vi "fpga_project_stable.vi"() -> ()   [LabVIEW 2019]
uses:
  <vilib>/Platform/TimedLoop/XDataNode/timing_clust.ctl
  <vilib>/Platform/TimedLoop/XDataNode/nitl_modes.ctl
  <vilib>/Platform/TimedLoop/XDataNode/wakeup.ctl
  <vilib>/rvi/eio/common/nirviEmuTemplateMethod_errors.vi
  <vilib>/rvi/Emulation/niFpgaSctlEmulationGetInTimedLoop.vi
  <vilib>/rvi/Emulation/niFpgaEmulationReportErrorSimple.vi
  <vilib>/rvi/Emulation/niFpgaGetClockAttributes.vi
  <vilib>/rvi/Emulation/niFpgaCriticalErrorInLSC.vi
  <vilib>/eio/EIONode/EIONode.xnode
  <vilib>/eio/EIOMethodNode/EIOMethodNode.xnode
  <vilib>/platform/TimedLoop/XDataNode/XDataNode.xnode
  <vilib>/Platform/TimedLoop/XDataNode/XDNodeRunTimeDep.lvlib
panel:
  out "SDA":bool
  out "ACK":bool
  in  "add + read bite":u8 format="%x"
  in  "register":u8 format="%x"
  in  "adresse + Write":u8 format="%x"
  out "adress + READ":bool[](array[boolean])
  out "DATA":u8 format="%b"
  out "DATA":bool[](array[boolean])
  out "register adress":bool[](array[boolean])
  out "Adresse + command byte":bool[](array[boolean])
  # "51"
  # "50"
  # "expected data :"
  # "00110011"
  # "15"
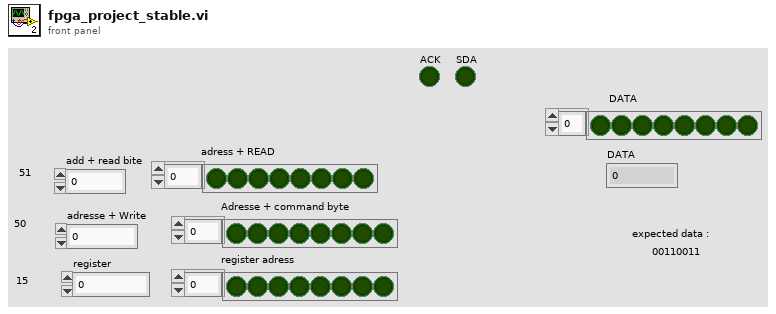
[diagram p1: front panel]
types:
  T1 = typedef "XDNodeRunTimeDep.lvlib/timing_clust.ctl" = cluster{"Expected End [f-1]":u64, "Actual End [f-1]":u64, "Finished Late? [f-1]":bool, "Expected End [i-1]":u64, "Actual End [i-1]":u64, "Finished Late? [i-1]":bool, "Expected Start [i]":u64, "Actual Start [i]":u64, "Expected Start [f]":u64, "Actual Start [f]":u64, "Source Name":string, "Structure Name":string, "Period":i64, "Deadline":i64, "Offset":i64, "Start":i64, "Priority":i32, "Timeout":i32, "Mode":T2, "Wakeup Reason":T3, "Error":errorcluster, "Source Type":string, "Secondary Source Type":string, "Global End Time":u64, "Global Start Time":u64, "Frame Duration":u64, "Iteration Duration":u64, "Assigned CPU":i32, "I/O Scan Engine Mode":u32}
  T2 = typedef "XDNodeRunTimeDep.lvlib/nitl_modes.ctl" = enum32{"No Change", "Process missed periods, maintain original phase", "Discard missed periods, maintain original phase", "Process missed periods, ignore original phase", "Discard missed periods, ignore original phase"}
  T3 = typedef "XDNodeRunTimeDep.lvlib/wakeup.ctl" = enum32{"Normal", "Aborted", "Asynchronous wakeup", "Timing source error", "Timed loop error", "Timeout"}
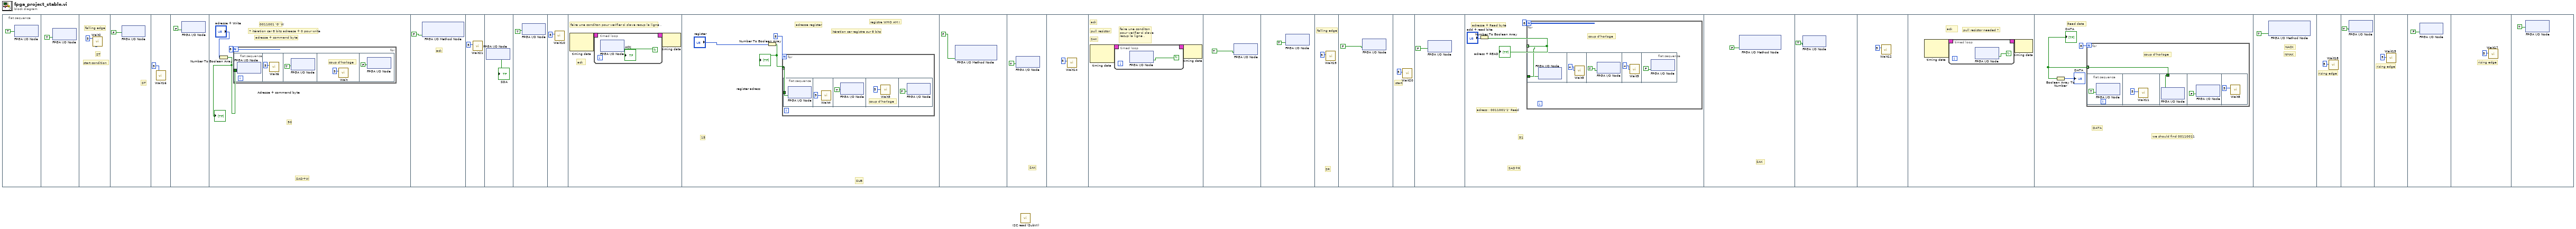
[diagram p0: block diagram]
diagram:
  n1 = flat-sequence {
    frame #0 {
      n2 = xnode "FPGA I/O Node"("SDA"=TRUE) -> ()  [unwired: 1 in, 1 out]
    }
    frame #1 {
      n3 = xnode "FPGA I/O Node"("SCL"=TRUE) -> ()  [unwired: 1 in, 1 out]
    }
    frame #2 {
      # "ST"
      # "start condition"
      # "falling edge"
      n4 = call "Wait2"("Count(Ticks)"=u32 5) -> ()  [unwired: 1 out]
    }
    frame #3 {
      # "ST"
      n5 = xnode "FPGA I/O Node"("SDA"=FALSE) -> ()  [unwired: 1 in, 1 out]
    }
    frame #4 {
      n6 = call "Wait16"("Count(Ticks)"=u32 5) -> ()  [unwired: 1 out]
    }
    frame #5 {
      n7 = xnode "FPGA I/O Node"("SCL"=FALSE) -> ()  [unwired: 1 in, 1 out]
    }
    frame #6 {
      # "50"
      # "SAD+W"
      # "7 itération car 8 bits adreese + 0 pour write"
      # "0011001 '0' W"
      # "adresse + command byte"
      n8 = Number To Boolean Array(number="adresse + Write") -> (Boolean array=w8:bool[])
      "Adresse + command byte" <- w8
      n9 = for {
        N: 8 -> [_]
        tunnel: w8 -> [w10] mode=indexing
        n10 = flat-sequence {
          tunnel: w10 -> [w11]
          frame #0 {
            n11 = xnode "FPGA I/O Node"("SDA"=w11) -> ()  [unwired: 1 in, 1 out]
          }
          frame #1 {
            n12 = call "Wait6"("Count(Ticks)"=u32 5) -> ()  [unwired: 1 out]
          }
          frame #2 {
            n13 = xnode "FPGA I/O Node"("SCL"=TRUE) -> ()  [unwired: 1 in, 1 out]
          }
          frame #3 {
            # "coup d'horloge"
            n14 = call "Wait"("Count(Ticks)"=u32 5) -> ()  [unwired: 1 out]
          }
          frame #4 {
            n15 = xnode "FPGA I/O Node"("SCL"=FALSE) -> ()  [unwired: 1 in, 1 out]
          }
        }
      }
    }
    frame #7 {
      # "ack"
      n16 = xnode "FPGA I/O Method Node"("Enable"=FALSE) -> ()  [unwired: 1 in, 1 out]
    }
    frame #8 {
      n17 = call "Wait21"("Count(Ticks)"=u32 5) -> ()  [unwired: 1 out]
    }
    frame #9 {
      n18 = xnode "FPGA I/O Node"() -> ("SDA"=→"SDA":bool)  [unwired: 1 in, 1 out]
    }
    frame #10 {
      n19 = xnode "FPGA I/O Node"("SCL"=TRUE) -> ()  [unwired: 1 in, 1 out]
    }
    frame #11 {
      n20 = call "Wait10"("Count(Ticks)"=u32 5) -> ()  [unwired: 1 out]
    }
    frame #12 {
      # "ack"
      # "faire une conditon pour verifier si slave recup la ligne ."
      n21 = node-c288() -> (w22:T1)  [unwired: 2 in]
      n22 = timed-loop {
        timing: w22 -> [_]
        timing-out: [_] -> w21
        stop <- w23 continue-if-true
        n23 = xnode "FPGA I/O Node"() -> ("SDA"=w23:bool)  [unwired: 1 in, 1 out]
        "ACK" <- w23
      }
      n24 = node-c288(w21) -> ()  [unwired: 1 out]
    }
    frame #13 {
      # "15"
      # "registre WHO AM I"
      # "itération car registre sur 8 bits"
      # "SUB"
      # "adresse register"
      n25 = Number To Boolean Array(number="register") -> (Boolean array=w30:bool[])
      "register adress" <- w30
      n26 = for {
        N: 8 -> [_]
        tunnel: w30 -> [w31] mode=indexing
        n27 = flat-sequence {
          tunnel: w31 -> [w32]
          frame #0 {
            n28 = xnode "FPGA I/O Node"("SDA"=w32) -> ()  [unwired: 1 in, 1 out]
          }
          frame #1 {
            n29 = call "Wait4"("Count(Ticks)"=u32 5) -> ()  [unwired: 1 out]
          }
          frame #2 {
            n30 = xnode "FPGA I/O Node"("SCL"=TRUE) -> ()  [unwired: 1 in, 1 out]
          }
          frame #3 {
            # "coup d'horloge"
            n31 = call "Wait3"("Count(Ticks)"=u32 5) -> ()  [unwired: 1 out]
          }
          frame #4 {
            n32 = xnode "FPGA I/O Node"("SCL"=FALSE) -> ()  [unwired: 1 in, 1 out]
          }
        }
      }
    }
    frame #14 {
      n33 = xnode "FPGA I/O Method Node"("Enable"=FALSE) -> ()  [unwired: 1 in, 1 out]
    }
    frame #15 {
      # "SAK"
      n34 = xnode "FPGA I/O Node"("SCL"=TRUE) -> ()  [unwired: 1 in, 1 out]
    }
    frame #16 {
      n35 = call "Wait14"("Count(Ticks)"=u32 5) -> ()  [unwired: 1 out]
    }
    frame #17 {
      # "SAK"
      # "ack"
      # "faire une conditon pour verifier si slave recup la ligne ."
      # "pull resistor"
      n36 = node-c288() -> (w41:T1)  [unwired: 2 in]
      n37 = timed-loop {
        timing: w41 -> [_]
        timing-out: [_] -> w40
        stop <- w42 continue-if-true
        n38 = xnode "FPGA I/O Node"() -> ("SDA"=w42:bool)  [unwired: 1 in, 1 out]
      }
      n39 = node-c288(w40) -> ()  [unwired: 1 out]
    }
    frame #18 {
      n40 = xnode "FPGA I/O Node"("SDA"=TRUE) -> ()  [unwired: 1 in, 1 out]
    }
    frame #19 {
      n41 = xnode "FPGA I/O Node"("SCL"=TRUE) -> ()  [unwired: 1 in, 1 out]
    }
    frame #20 {
      # "SR"
      # "falling edge"
      n42 = call "Wait19"("Count(Ticks)"=u32 5) -> ()  [unwired: 1 out]
    }
    frame #21 {
      n43 = xnode "FPGA I/O Node"("SDA"=FALSE) -> ()  [unwired: 1 in, 1 out]
    }
    frame #22 {
      # "start"
      n44 = call "Wait20"("Count(Ticks)"=u32 5) -> ()  [unwired: 1 out]
    }
    frame #23 {
      n45 = xnode "FPGA I/O Node"("SCL"=FALSE) -> ()  [unwired: 1 in, 1 out]
    }
    frame #24 {
      # "51"
      # "SAD+R"
      # "adress : 0011001'1' Read"
      # "adresse + Read byte"
      n46 = Number To Boolean Array(number="add + read bite") -> (Boolean array=w55:bool[])
      "adress + READ" <- w55
      n47 = for {
        N: 8 -> [_]
        tunnel: w55 -> [w56] mode=indexing
        # "coup d'horloge"
        n48 = flat-sequence {
          tunnel: w56 -> [w57]
          frame #0 {
            n49 = xnode "FPGA I/O Node"("SDA"=w57) -> ()  [unwired: 1 in, 1 out]
          }
          frame #1 {
            n50 = call "Wait5"("Count(Ticks)"=u32 4) -> ()  [unwired: 1 out]
          }
          frame #2 {
            n51 = xnode "FPGA I/O Node"("SCL"=TRUE) -> ()  [unwired: 1 in, 1 out]
          }
          frame #3 {
            n52 = call "Wait9"("Count(Ticks)"=u32 4) -> ()  [unwired: 1 out]
          }
          frame #4 {
            n53 = xnode "FPGA I/O Node"("SCL"=FALSE) -> ()  [unwired: 1 in, 1 out]
          }
        }
      }
    }
    frame #25 {
      # "SAK"
      n54 = xnode "FPGA I/O Method Node"("Enable"=FALSE) -> ()  [unwired: 1 in, 1 out]
    }
    frame #26 {
      n55 = xnode "FPGA I/O Node"("SCL"=TRUE) -> ()  [unwired: 1 in, 1 out]
    }
    frame #27 {
      n56 = call "Wait12"("Count(Ticks)"=u32 5) -> ()  [unwired: 1 out]
    }
    frame #28 {
      # "ack"
      # "pull resistor needed ?"
      n57 = node-c288() -> (w66:T1)  [unwired: 2 in]
      n58 = timed-loop {
        timing: w66 -> [_]
        timing-out: [_] -> w65
        stop <- w67 continue-if-true
        n59 = xnode "FPGA I/O Node"() -> ("SDA"=w67:bool)  [unwired: 1 in, 1 out]
      }
      n60 = node-c288(w65) -> ()  [unwired: 1 out]
    }
    frame #29 {
      # "we should find 00110011"
      # "DATA"
      # "Read data"
      n61 = for {
        N: 8 -> [_]
        tunnel: [w75] -> w73 mode=indexing
        # "coup d'horloge"
        n62 = flat-sequence {
          tunnel: [w78] -> w75
          frame #0 {
            n63 = xnode "FPGA I/O Node"("SCL"=TRUE) -> ()  [unwired: 1 in, 1 out]
          }
          frame #1 {
            n64 = call "Wait11"("Count(Ticks)"=u32 5) -> ()  [unwired: 1 out]
          }
          frame #2 {
            n65 = xnode "FPGA I/O Node"() -> ("SDA"=w78:bool)  [unwired: 1 in, 1 out]
          }
          frame #3 {
            n66 = xnode "FPGA I/O Node"("SCL"=FALSE) -> ()  [unwired: 1 in, 1 out]
          }
          frame #4 {
            n67 = call "Wait8"("Count(Ticks)"=u32 5) -> ()  [unwired: 1 out]
          }
        }
      }
      "DATA" <- w73
      n68 = Boolean Array To Number(Boolean array=w73) -> (number=→"DATA":u8)
    }
    frame #30 {
      # "NMAK"
      # "NACK"
      n69 = xnode "FPGA I/O Method Node"("Enable"=TRUE) -> ()  [unwired: 1 in, 1 out]
    }
    frame #31 {
      # "rising edge"
      n70 = call "Wait18"("Count(Ticks)"=u32 5) -> ()  [unwired: 1 out]
    }
    frame #32 {
      n71 = xnode "FPGA I/O Node"("SCL"=TRUE) -> ()  [unwired: 1 in, 1 out]
    }
    frame #33 {
      # "rising edge"
      n72 = call "Wait15"("Count(Ticks)"=u32 5) -> ()  [unwired: 1 out]
    }
    frame #34 {
      n73 = xnode "FPGA I/O Node"("SDA"=FALSE) -> ()  [unwired: 1 in, 1 out]
    }
    frame #35 {
      # "rising edge"
      n74 = call "Wait17"("Count(Ticks)"=u32 5) -> ()  [unwired: 1 out]
    }
    frame #36 {
      n75 = xnode "FPGA I/O Node"("SDA"=TRUE) -> ()  [unwired: 1 in, 1 out]
    }
  }
  n76 = call "I2C read (SubVI).vi"() -> ()  [unwired: 11 in, 1 out]
